vi "GetRunningServerInfo.vi"(0 "New Server":T2={"vi name"="", "queue"=refnum, "ROS"={"topic port"=0, "Node"="", "topic"="", "type"="", "node port"=0, "error "={"status"=FALSE, "code"=0, "source"=""}, "Direction"=enum."Node", "Update (ms)"=1, "FIFO size"=1}, "notifier"=refnum, "FIFO"=refnum, "This VI"=refnum, "MyState"=enum."No Connection"}, 1 "Task":T1(ring)=enum."Get Info") -> (2 "Status":T5[](array[typedef]), 3 "servers":T2[](array[typedef]), 4 "Topics":string[](array[string]))   [LabVIEW 2012]
uses:
  <userlib>/ROSforLV/ROS/Code/Console/Servers/ServerSubs/MyState.ctl
  <userlib>/ROSforLV/ROS/Code/Console/Servers/ServerSubs/ServoInfo.ctl
  <userlib>/ROSforLV/ROS/Code/SubVIs/_ROSControl.ctl
  <userlib>/ROSforLV/ROS/Code/SubVIs/_ROSDirection.ctl
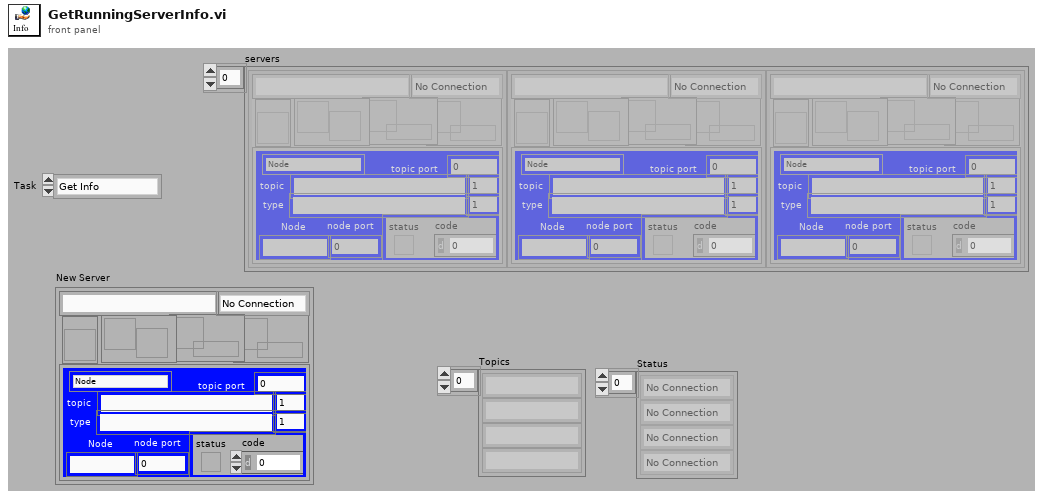
[diagram p1: front panel]
types:
  T1 = enum16{"Add Server", "Clear Server", "Clear All", "Get Info", "GetPanelInfo", "ChangeState"}
  T2 = typedef "ServoInfo.ctl" = cluster{"vi name":string, "queue":refnum<queue>, "ROS":T3, "notifier":refnum<notifier>, "FIFO":refnum<queue>, "This VI":refnum<vi>, "MyState":T5}
  T3 = typedef "_ROSControl.ctl" = cluster{"topic port":u16, "Node":string, "topic":string, "type":string, "node port":u16, "error ":errorcluster, "Direction":T4, "Update (ms)":u16, "FIFO size":u16}
  T4 = typedef "_ROSDirection.ctl" = enum16{"Node", "Publisher", "Subscriber", "ServiceClient", "ServiceProvider"}
  T5 = typedef "MyState.ctl" = enum16{"No Connection", "Registered", "Connected", "Close"}
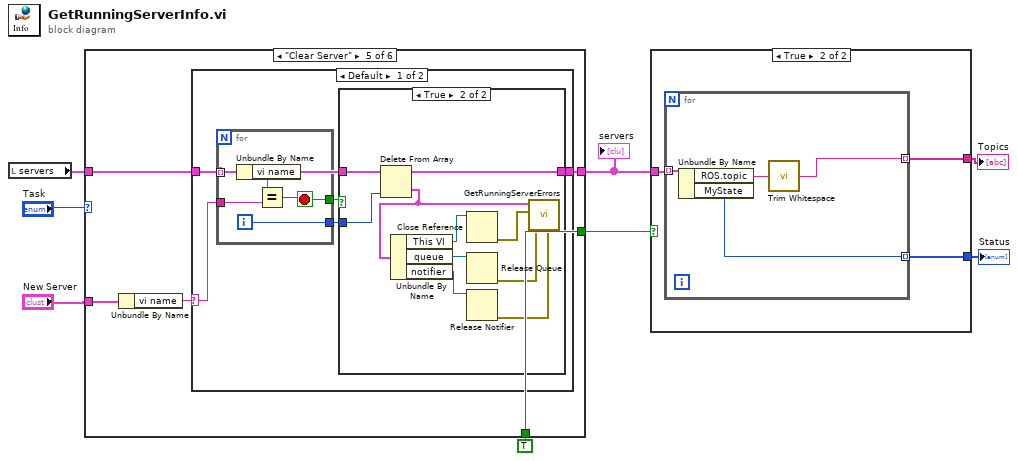
[diagram p0: block diagram]
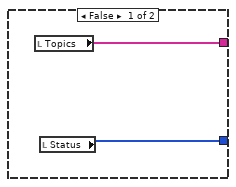
[diagram p2: hidden frame]
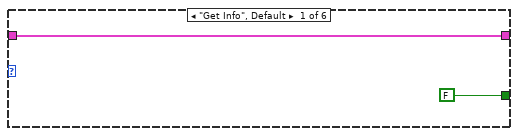
[diagram p3: hidden frame]
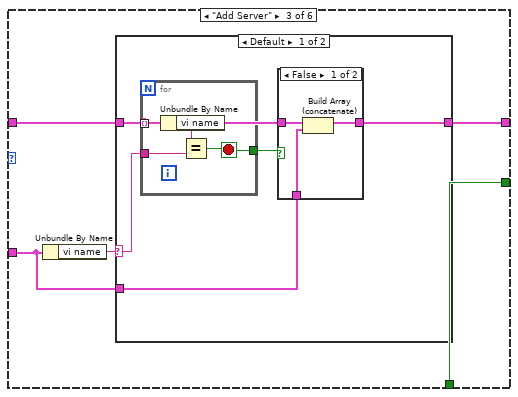
[diagram p5: hidden frame]
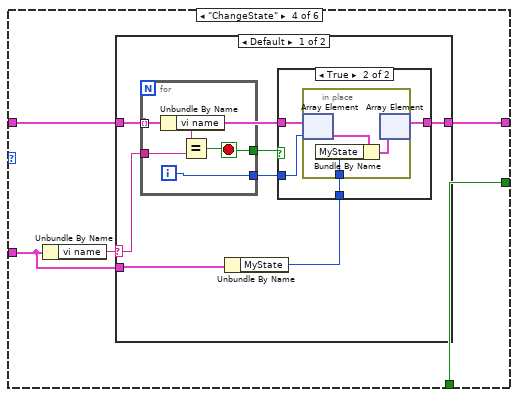
[diagram p8: hidden frame]
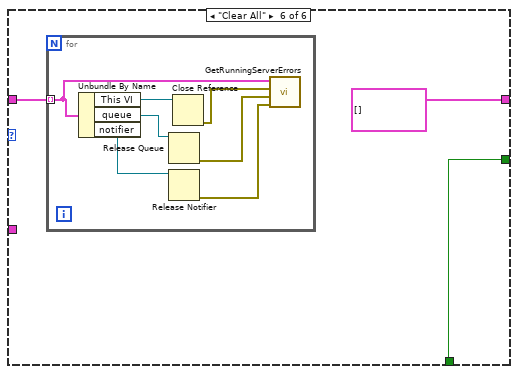
[diagram p13: hidden frame]
diagram:
  n1 = local read "servers"() -> (w2:T2[])
  n2 = case shown="\"Clear Server\"" "Task" {
    tunnel: w2 -> [w10 w12 w16 w35 w61 w87]
    tunnel: "New Server" -> [_ _ w14 w33 w59 _]
    tunnel: [w10 w12 w15 w34 w60 T2[] [] ("servers")] -> w1
    tunnel: [FALSE ("First Call?: T/F") w11 w13 w32 w58 w86] -> w6
    tunnel: TRUE ("First Call?: T/F") -> [_ w11 w13 w32 w58 w86]
    frame "Get Info", Default {
    }
    frame "GetPanelInfo" {
    }
    frame "Add Server" {
      n3 = Unbundle By Name(w14) -> ("vi name"=w17:string)
      n4 = case shown="Default" w17 {
        selector: w17 -> [w22 _]
        tunnel: [w20 w31] -> w15
        tunnel: w16 -> [w19 w31]
        tunnel: w14 -> [w18 _]
        frame Default {
          n5 = for {
            tunnel: w19 -> [w30] mode=indexing
            tunnel: w22 -> [w28]
            tunnel: [w27] -> w21
            stop <- w27 stop-if-true
            n6 = Unbundle By Name(w30) -> ("vi name"=w29:string)
            n7 = Equal?(x=w29, y=w28) -> (x = y?=w27:bool)
          }
          n8 = case shown="False" w21 {
            tunnel: [w23 w26] -> w20
            tunnel: w19 -> [w25 w26]
            tunnel: w18 -> [w24 _]
            frame False {
              n9 = Build Array (concatenate)(w25, w24) -> (w23:T2[])
            }
            frame True {
            }
          }
        }
        frame "" {
        }
      }
    }
    frame "ChangeState" {
      n10 = Unbundle By Name(w33) -> ("vi name"=w36:string)
      n11 = case shown="Default" w36 {
        selector: w36 -> [w43 _]
        tunnel: [w41 w57] -> w34
        tunnel: w35 -> [w40 w57]
        tunnel: w33 -> [w38 _]
        frame Default {
          n12 = for {
            tunnel: w40 -> [w56] mode=indexing
            tunnel: w43 -> [w54]
            tunnel: [w53] -> w42
            tunnel: [w52] -> w39
            i -> [w52]
            stop <- w53 stop-if-true
            n13 = Unbundle By Name(w56) -> ("vi name"=w55:string)
            n14 = Equal?(x=w55, y=w54) -> (x = y?=w53:bool)
          }
          n15 = Unbundle By Name(w38) -> ("MyState"=w37:T5)
          n16 = case shown="True" w42 {
            tunnel: [w44 w46] -> w41
            tunnel: w40 -> [w44 w48]
            tunnel: w39 -> [_ w47]
            tunnel: w37 -> [_ w45]
            frame False {
            }
            frame True {
              n17 = in-place {
                in-place-border: w45 -> [w49]
                n18 = in-place-array #1(w48, w47) -> (w51:T2)
                n19 = Bundle By Name(cluster=w51, "MyState"=w49) -> (w50:T2)
                n20 = in-place-array #1(w50) -> (w46:T2[])  [unwired: 1 out]
              }
            }
          }
        }
        frame "" {
        }
      }
    }
    frame "Clear Server" {
      n21 = Unbundle By Name(w59) -> ("vi name"=w62:string)
      n22 = case shown="Default" w62 {
        selector: w62 -> [w67 _]
        tunnel: [w65 w84] -> w60
        tunnel: w61 -> [w64 w84]
        frame Default {
          n23 = for {
            tunnel: w64 -> [w83] mode=indexing
            tunnel: w67 -> [w81]
            tunnel: [w80] -> w66
            tunnel: [w79] -> w63
            i -> [w79]
            stop <- w80 stop-if-true
            n24 = Unbundle By Name(w83) -> ("vi name"=w82:string)
            n25 = Equal?(x=w82, y=w81) -> (x = y?=w80:bool)
          }
          n26 = case shown="True" w66 {
            tunnel: [w68 w76] -> w65
            tunnel: w64 -> [w68 w77]
            tunnel: w63 -> [_ w78]
            frame False {
            }
            frame True {
              n27 = Delete From Array(array=w77, index=w78) -> (deleted portion=w69:T2, array with subset deleted=w76:T2[])  [unwired: 1 in]
              n28 = Unbundle By Name(w69) -> ("This VI"=w73:refnum<vi>, "queue"=w75:refnum<queue>, "notifier"=w74:refnum<notifier>)
              n29 = Close Reference(reference=w73) -> (error out=w72:errorcluster)  [unwired: 1 in]
              n30 = Release Queue(queue=w75) -> (error out=w71:errorcluster)  [unwired: 2 in, 2 out]
              n31 = Release Notifier(notifier=w74) -> (error out=w70:errorcluster)  [unwired: 2 in, 2 out]
              n32 = call <userlib>:"GetRunningServerErrors.vi"("error release notification"=w70, "error release queue"=w71, "error close reference"=w72, "server"=w69) -> ()  [unwired: 8 in]
            }
          }
        }
        frame "" {
        }
      }
    }
    frame "Clear All" {
      n33 = for {
        tunnel: w87 -> [w88] mode=indexing
        n34 = Unbundle By Name(w88) -> ("This VI"=w94:refnum<vi>, "queue"=w93:refnum<queue>, "notifier"=w92:refnum<notifier>)
        n35 = Release Queue(queue=w93) -> (error out=w90:errorcluster)  [unwired: 2 in, 2 out]
        n36 = Release Notifier(notifier=w92) -> (error out=w89:errorcluster)  [unwired: 2 in, 2 out]
        n37 = Close Reference(reference=w94) -> (error out=w91:errorcluster)  [unwired: 1 in]
        n38 = call <userlib>:"GetRunningServerErrors.vi"("error release notification"=w89, "error release queue"=w90, "error close reference"=w91, "server"=w88) -> ()  [unwired: 8 in]
      }
    }
  }
  "servers" <- w1
  n39 = case shown="True" w6 {
    tunnel: w1 -> [_ w99]
    tunnel: [w95 w98] -> w4
    tunnel: [w96 w97] -> w3
    frame False {
      n40 = local read "Topics"() -> (w95:string[])
      n41 = local read "Status"() -> (w96:T5[])
    }
    frame True {
      n42 = for {
        tunnel: w99 -> [w101] mode=indexing
        tunnel: [w103] -> w98 mode=indexing
        tunnel: [w100] -> w97 mode=indexing
        n43 = Unbundle By Name(w101) -> ("ROS.topic"=w102:string, "MyState"=w100:T5)
        n44 = call <vilib>:"Trim Whitespace.vi"("string"=w102) -> ("trimmed string"=w103:string)  [unwired: 1 in]
      }
    }
  }
  "Topics" <- w4
  "Status" <- w3
